vi "Connection Retries--constant.vi"() -> (3 "Retries":i32=10)   [LabVIEW 2024, in "CTIWrapper.lvlib"]
uses:
  CTIWrapper.lvlib
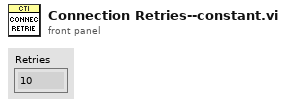
[diagram p1: front panel]
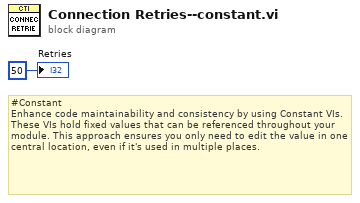
[diagram p0: block diagram]
diagram:
  # "#Constant\nEnhance code maintainability and consistency by using Constant VIs. These VIs hold fixed values that can be referenced throughout your module. This approach ensures you only need to edit the value in one central location, even if it's used in multiple places."
  "Retries" <- 50 ("Retries")
